vi "MultiChannelFeedbackCooling_aod_feedback(Host).vi"(5 "RIO Device":T2="RIO0") -> ()   [LabVIEW 2014]
doc: "This VI will will initialize the FPGA VI and then continually read and convert single point values from 4 channels of an analog input module."
uses:
  <vilib>/userdefined/High Color/nirio_resource_hc.ctl
  <vilib>/rvi/Analysis/host/Butterworth/config/Butterworth Filter Order.ctl
  <vilib>/rvi/Analysis/host/Butterworth/config/Butterworth Filter Type.ctl
  <vilib>/FPGAPlugInAG/PXI-7854R/niLvFpga_Open_PXI-7854R.vi
  <vilib>/FPGAPlugInAG/PXI-7854R/niLvFpga_Run_PXI-7854R.vi
  <vilib>/Utility/error.llb/Error Cluster From Error Code.vi
  <vilib>/rvi/errors/niLvFpgaAdjustHostInterfaceError.vi
  <vilib>/rvi/Analysis/host/Butterworth/config/BwScaledCoefficients.vi
  <vilib>/FPGAPlugInAG/PXI-7854R/niLvFpga_Close_PXI-7854R.vi
  <vilib>/rvi/interface/nirviOpenFPGA/nirviOpenFPGA.xnode
  FPGA Bitfiles/MultiChannelFeed_FPGATarget_MultiChannelfFee_xkdZYBc6TtU.lvbitx
  <vilib>/rvi/interface/nirviMethod/nirviMethod.xnode
  <vilib>/rvi/interface/nirviReadWriteControl/nirviReadWriteControl.xnode
  <vilib>/rvi/Analysis/host/Butterworth/XNode/ButterworthCoefficients.xnode
  <vilib>/rvi/interface/nirviCloseFPGA/nirviCloseFPGA.xnode
  <vilib>/rvi/Analysis/host/Public/NI_FpgaMspHost.lvlib
  NiFpgaLv.dll
panel:
  in  "bits per pi 2":i16=100
  in  "Reset Counter":bool
  in  "counter offset":u32
  in  "c3_delay_mult":i16=-1
  in  "c3_mult":i16=1
  in  "c2_delay_mult":i16=-1
  in  "c2_mult":i16=-1
  in  "c1_delay_mult":i16=1
  in  "c1_mult":i16=-1
  in  "c0_delay_mult":i16=1
  in  "c0_mult":i16=1
  in  "pg_img":fxp<+/-,24,12>
  in  "dg_img":fxp<+/-,24,12>
  in  "ig_img":fxp<+/-,24,6>
  in  "setpt_img":i16=3000
  in  "Upper lim_img":fxp<+/-,16,16>=1000.0
  in  "Lower lim_img":fxp<+/-,16,16>=-1000.0
  in  "output offset_img":i16
  out "Phi_filt h/lpf":dbl(graph)=-1.7364501953125
  in  "phase_hpf":dbl=2.0
  in  "Use phase hpf?":bool=TRUE
  in  "phase offset":i16
  in  "phase discont_neg":fxp<+/-,24,12>=-1.0
  in  "phase discont_pos":fxp<+/-,24,12>=1.0
  in  "Use phase lpf?":bool
  in  "phase_lpf":dbl=10000.0
  in  "Host Update Rate (msec)":dbl=1.0 format="%#_13g"
  in  "ADC Loop Timer (usec)":u32=5
  out "Phi":dbl(graph)=-0.99530029296875
  in  "Reset Phi":bool
  out "Phi Full":dbl(graph)=8.9061279296875
  in  "Bits Per Pi":i16=2000
  in  "change pars 3":bool
  in  "Mixing Level":i16=32767
  in  "Save gain setting?":bool
  in  "Step Y Gain?":bool
  in  "Enum 2":enum16{"Increase Y Gain", "Decrease Y Gain"}(ring)=enum."Decrease Y Gain"
  in  "Step X Gain?":bool
  in  "Enum":enum16{"Increase X Gain", "Decrease X Gain"}(ring)=enum."Decrease X Gain"
  in  "Ygain":T1(ring)=enum."20"
  in  "Xgain":T1(ring)=enum."20"
  in  "Change Post-Mixing Gain?":bool
  in  "Ref AOM Lvl":i16=-32768
  in  "Piezo Z":i16=-32768
  in  "power setpt":i16=7000
  in  "Upper lim pow":fxp<+/-,16,16>=10000.0
  in  "Lower lim pow":fxp<+/-,16,16>=-10000.0
  in  "hp freq pow":dbl=5000.0
  in  "lp freq pow":dbl=5000.0
  in  "Use_PID2_power":bool
  in  "hp freq 1":dbl=2200.0
  in  "hp freq 0":dbl=2200.0
  in  "lp freq 0":dbl=2200.0
  in  "DC offset 0":i16
  in  "Lower lim 0":fxp<+/-,16,16>=-1000.0
  in  "Upper lim 0":fxp<+/-,16,16>=1000.0
  in  "Dg 0":fxp<+/-,24,12>=-0.10009765625
  in  "Bead setpt 0":i16
  in  "change pars":bool
  in  "hp freq 2":dbl=1100.0
  in  "lp freq 1":dbl=2200.0
  in  "lp freq 2":dbl=1100.0
  in  "ramp power":bool
  in  "End value power":i16=1600
  in  "Step power":i16=5
  in  "Delay Time (s) power":dbl=0.01 caption="Delay Time (s)"
  in  "?":u16(ring)=2 items=["Both", "AOD", "Bead"]
  in  "?":u16(ring)=2 items=["Both", "AOD", "Bead"]
  in  "?":u16(ring) items=["Both", "AOD", "Bead"]
  in  "?":u16(ring)=2 items=["Both", "AOD", "Bead"]
  in  "?":u16(ring)=1 items=["Both", "AOD", "Bead"]
  in  "?":u16(ring)=2 items=["Both", "AOD", "Bead"]
  in  "Pg d2":fxp<+/-,24,12>=-6.0
  in  "Ig d2":fxp<+/-,24,6>=-0.7999992370605469
  in  "Dg d2":fxp<+/-,24,12>
  in  "Ig 2":fxp<+/-,24,6>
  in  "DC offset 2":i16=-16750
  in  "Lower lim 2":fxp<+/-,16,16>=-2000.0
  in  "Upper lim 2":fxp<+/-,16,16>=2000.0
  in  "Dg 2":fxp<+/-,24,12>=-1.0
  in  "Pg 2":fxp<+/-,24,12>=-0.10009765625
  in  "Bead setpt 2":i16=-2800
  in  "change pars 2":bool
  in  "change pars 1":bool
  in  "DC offset 1":i16
  in  "Lower lim 1":fxp<+/-,16,16>=-1000.0
  in  "Upper lim 1":fxp<+/-,16,16>=1000.0
  in  "Dg 1":fxp<+/-,24,12>=-0.10009765625
  in  "Bead setpt 1":i16
  out "Tot feedback + DC, Ch2":i16(graph)=-16644
  out "Individual feedback, Ch2":cluster{"fb_0":i16, "fb_d0":i16}(graph)={"fb_0"=108, "fb_d0"=108}
  out "AI2":cluster{"AI2":i16, "AI5":i16}(graph)={"AI2"=-3445, "AI5"=-3445}
  out "Tot feedback + DC, Ch1":i16(graph)=14
  out "Individual feedback, Ch1":cluster{"fb_0":i16, "fb_d0":i16}(graph)={"fb_0"=14, "fb_d0"=14}
  out "AI1":cluster{"AI1":i16, "AI4":i16}(graph)={"AI1"=1858, "AI4"=1858}
  out "Tot feedback + DC, Ch0":i16(graph)=17
  out "Individual feedback, Ch0":cluster{"fb_0":i16, "fb_d0":i16}(graph)={"fb_0"=17, "fb_d0"=17}
  out "AI0":cluster{"AI0":i16, "AI3":i16}(graph)={"AI0"=12513, "AI3"=12513}
  in  "stop":bool
  # "FPGA feedback GUI"
  # "PID controls, X (ch 0):"
  # "Gain Control"
  # "Pre-Mixing Gain"
  # "Ref Mixing Level"
  # "PID controls, Y (ch 1):"
  # "Bead feedback:"
  # "Post-Mixing Gain"
  # "Backscatter Interferometer Settings"
  # "Phase wrapping"
  # "Bead feedback:"
  # "PID controls, Z (ch 2):"
  # "Bead feedback:"
  # "AOD feeback:"
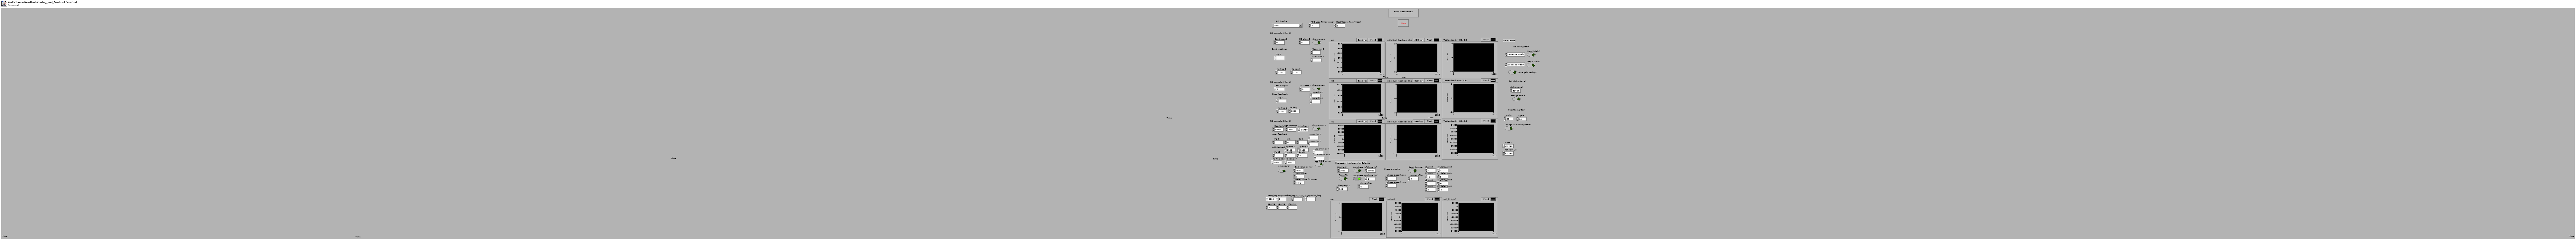
[diagram p1: front panel]
types:
  T1 = enum16{"1", "2", "4", "8", "10", "20", "40", "80", "100", "200", "400", "800"}
  T2 = typedef "nirio_resource_hc.ctl" = tag
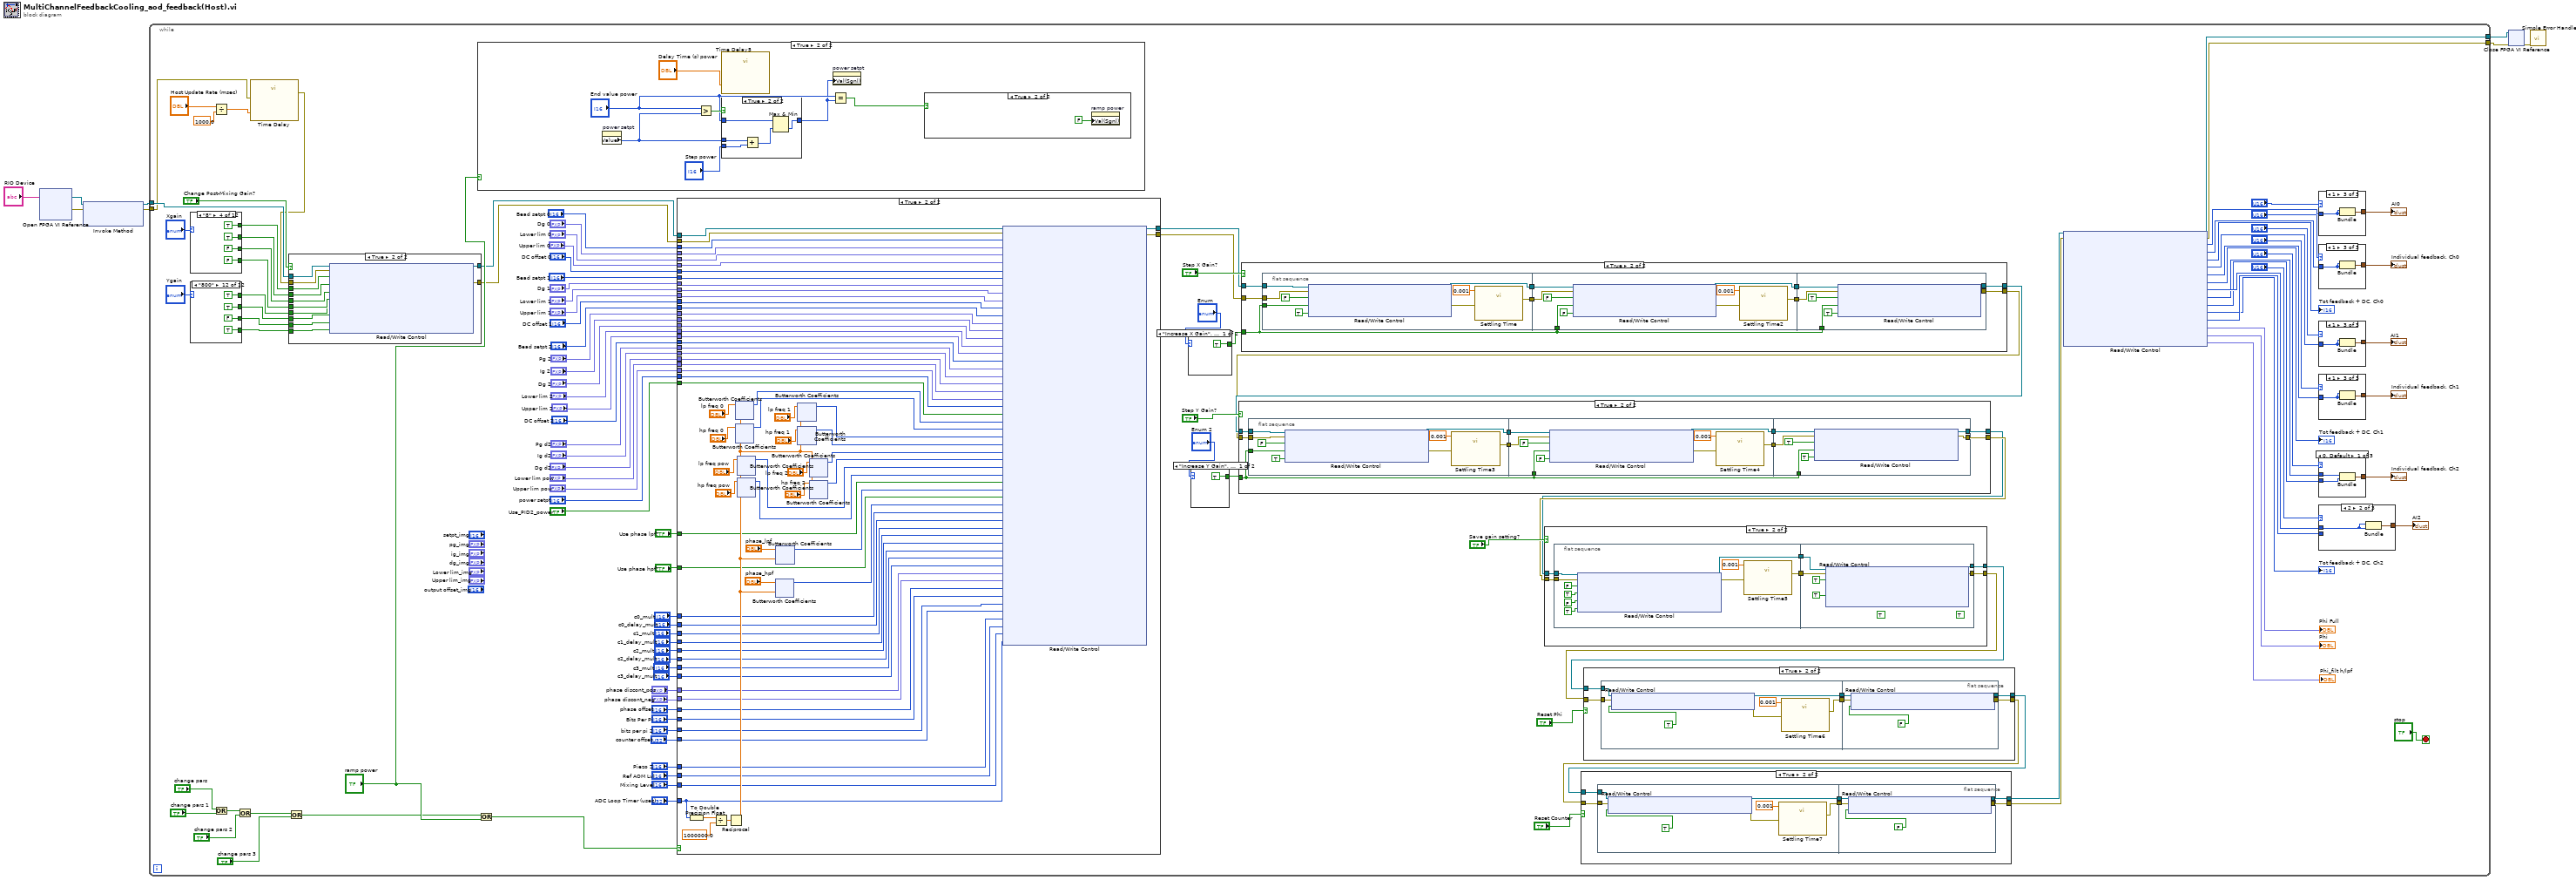
[diagram p0: block diagram]
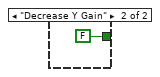
[diagram p6: hidden frame]
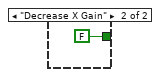
[diagram p8: hidden frame]
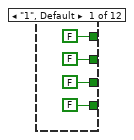
[diagram p9: hidden frame]
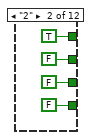
[diagram p10: hidden frame]
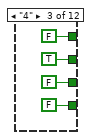
[diagram p11: hidden frame]
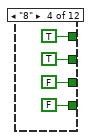
[diagram p12: hidden frame]
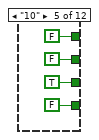
[diagram p13: hidden frame]
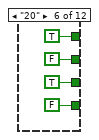
[diagram p14: hidden frame]
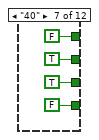
[diagram p15: hidden frame]
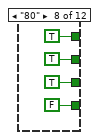
[diagram p16: hidden frame]
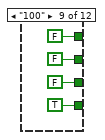
[diagram p17: hidden frame]
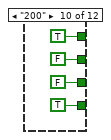
[diagram p18: hidden frame]
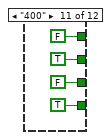
[diagram p19: hidden frame]
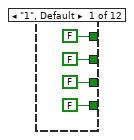
[diagram p20: hidden frame]
diagram:
  n1 = xnode "Open FPGA VI Reference"("resource name"="RIO Device") -> ("FPGA VI Reference Out"=w3:refnum<k20>, "error out"=w2:errorcluster)  [unwired: 1 in]
  n2 = xnode "Invoke Method"("FPGA VI Reference In"=w3, "error in"=w2) -> ("FPGA VI Reference Out"=w5:refnum<k20>, "error out"=w4:errorcluster)  [unwired: 1 in]
  n3 = while {
    tunnel: [w130] -> w8
    tunnel: w5 -> [w61]
    tunnel: w4 -> [w32]
    tunnel: [w129] -> w1
    stop <- "stop" stop-if-true
    n4 = case shown="\"8\"" "Xgain" {
      tunnel: [FALSE TRUE FALSE TRUE FALSE TRUE FALSE TRUE FALSE TRUE FALSE TRUE] -> w71
      tunnel: [FALSE FALSE TRUE TRUE FALSE FALSE TRUE TRUE FALSE FALSE TRUE TRUE] -> w70
      tunnel: [FALSE FALSE FALSE FALSE TRUE TRUE TRUE TRUE FALSE FALSE FALSE FALSE] -> w69
      tunnel: [FALSE FALSE FALSE FALSE FALSE FALSE FALSE FALSE TRUE TRUE TRUE TRUE] -> w68
      frame "1", Default {
      }
      frame "2" {
      }
      frame "4" {
      }
      frame "8" {
      }
      frame "10" {
      }
      frame "20" {
      }
      frame "40" {
      }
      frame "80" {
      }
      frame "100" {
      }
      frame "200" {
      }
      frame "400" {
      }
      frame "800" {
      }
    }
    n5 = case shown="\"800\"" "Ygain" {
      tunnel: [FALSE TRUE FALSE TRUE FALSE TRUE FALSE TRUE FALSE TRUE FALSE TRUE] -> w63
      tunnel: [FALSE FALSE TRUE TRUE FALSE FALSE TRUE TRUE FALSE FALSE TRUE TRUE] -> w64
      tunnel: [FALSE FALSE FALSE FALSE TRUE TRUE TRUE TRUE FALSE FALSE FALSE FALSE] -> w65
      tunnel: [FALSE FALSE FALSE FALSE FALSE FALSE FALSE FALSE TRUE TRUE TRUE TRUE] -> w66
      frame "1", Default {
      }
      frame "2" {
      }
      frame "4" {
      }
      frame "8" {
      }
      frame "10" {
      }
      frame "20" {
      }
      frame "40" {
      }
      frame "80" {
      }
      frame "100" {
      }
      frame "200" {
      }
      frame "400" {
      }
      frame "800" {
      }
    }
    n6 = Divide(x="Host Update Rate (msec)", y=1000.0) -> (x/y=w34:dbl)
    n7 = Or(x="change pars", y="change pars 1") -> (x .or. y?=w104:bool)
    n8 = Or(x=w104, y="change pars 2") -> (x .or. y?=w43:bool)
    n9 = call "Time Delay"("error in (no error)"=w32, "Delay Time (s)"=w34) -> ("error out"=w31:errorcluster)  [unwired: 9 in]
    n10 = case shown="True" "Change Post-Mixing Gain?" {
      tunnel: w71 -> [_ w380]
      tunnel: w70 -> [_ w379]
      tunnel: w69 -> [_ w378]
      tunnel: w68 -> [_ w377]
      tunnel: w66 -> [_ w376]
      tunnel: w65 -> [_ w375]
      tunnel: w64 -> [_ w374]
      tunnel: w63 -> [_ w373]
      tunnel: w31 -> [w367 w372]
      tunnel: [w367 w371] -> w62
      tunnel: w61 -> [w368 w370]
      tunnel: [w368 w369] -> w60
      frame False {
      }
      frame True {
        n11 = xnode "Read/Write Control"("FPGA VI Reference In"=w370, "error in"=w372, "XD0"=w380, "XD1"=w379, "XD2"=w378, "XD3"=w377, "YD0"=w373, "YD1"=w374, "YD2"=w375, "YD3"=w376) -> ("FPGA VI Reference Out"=w369:refnum<k20>, "error out"=w371:errorcluster)
      }
    }
    n12 = Or(x=w43, y="change pars 3") -> (x .or. y?=w30:bool)
    n13 = case shown="True" "ramp power" {
      frame False {
      }
      frame True {
        n14 = property on="power setpt" class="DigNum (strict)"() -> ("Value"=w382:i16)  [unwired: 2 in, 2 out]
        n15 = Greater?(x="End value power", y=w382) -> (0:w387:bool)
        n16 = call "Time Delay5"("Delay Time (s)"="Delay Time (s) power") -> ()  [unwired: 10 in, 1 out]
        n17 = case shown="True" w387 {
          tunnel: "End value power" -> [w390 w395]
          tunnel: w382 -> [w393 w398]
          tunnel: "Step power" -> [w392 w397]
          tunnel: [w389 w394] -> w381
          frame False {
            n18 = Subtract(x=w393, y=w392) -> (x-y=w391:i16)
            n19 = Max & Min(x=w390, y=w391) -> (max(x,y)=w389:i16)  [unwired: 1 out]
          }
          frame True {
            n20 = Add(x=w398, y=w397) -> (x+y=w396:i16)
            n21 = Max & Min(x=w395, y=w396) -> (min(x,y)=w394:i16)  [unwired: 1 out]
          }
        }
        n22 = property on="power setpt" class="DigNum (strict)"("Val(Sgnl)"=w381) -> ()  [unwired: 2 in, 2 out]
        n23 = Equal?(x="End value power", y=w381) -> (x = y?=w386:bool)
        n24 = case shown="True" w386 {
          frame False {
          }
          frame True {
            n25 = property on="ramp power" class="Bool (strict)"("Val(Sgnl)"=FALSE) -> ()  [unwired: 2 in, 2 out]
          }
        }
      }
    }
    n26 = Or(x=w30, y="ramp power") -> (x .or. y?=w80:bool)
    n27 = case shown="True" w80 {
      tunnel: w62 -> [w438 w502]
      tunnel: [w438 w510] -> w49
      tunnel: [w437 w509] -> w50
      tunnel: "Bead setpt 0" -> [_ w508]
      tunnel: "Dg 0" -> [_ w507]
      tunnel: "Upper lim 0" -> [_ w505]
      tunnel: "Lower lim 0" -> [_ w506]
      tunnel: "DC offset 0" -> [_ w504]
      tunnel: w60 -> [w437 w503]
      tunnel: "Bead setpt 1" -> [_ w501]
      tunnel: "Dg 1" -> [_ w500]
      tunnel: "Lower lim 1" -> [_ w499]
      tunnel: "Upper lim 1" -> [_ w498]
      tunnel: "DC offset 1" -> [_ w475]
      tunnel: "Bead setpt 2" -> [_ w497]
      tunnel: "Pg 2" -> [_ w496]
      tunnel: "Ig 2" -> [_ w477]
      tunnel: "Dg 2" -> [_ w495]
      tunnel: "Lower lim 2" -> [_ w494]
      tunnel: "Upper lim 2" -> [_ w493]
      tunnel: "DC offset 2" -> [_ w492]
      tunnel: "Pg d2" -> [_ w476]
      tunnel: "Ig d2" -> [_ w482]
      tunnel: "Dg d2" -> [_ w481]
      tunnel: "Use_PID2_power" -> [_ w485]
      tunnel: "Lower lim pow" -> [_ w478]
      tunnel: "Upper lim pow" -> [_ w479]
      tunnel: "power setpt" -> [_ w480]
      tunnel: "Piezo Z" -> [_ w453]
      tunnel: "Ref AOM Lvl" -> [_ w454]
      tunnel: "Mixing Level" -> [_ w455]
      tunnel: "Bits Per Pi" -> [_ w441]
      tunnel: "ADC Loop Timer (usec)" -> [_ w456]
      tunnel: "Use phase lpf?" -> [_ w460]
      tunnel: "phase discont_pos" -> [_ w444]
      tunnel: "phase discont_neg" -> [_ w443]
      tunnel: "phase offset" -> [_ w442]
      tunnel: "Use phase hpf?" -> [_ w458]
      tunnel: "c0_mult" -> [_ w452]
      tunnel: "c0_delay_mult" -> [_ w451]
      tunnel: "c1_mult" -> [_ w450]
      tunnel: "c1_delay_mult" -> [_ w449]
      tunnel: "c2_mult" -> [_ w448]
      tunnel: "c2_delay_mult" -> [_ w447]
      tunnel: "c3_mult" -> [_ w446]
      tunnel: "c3_delay_mult" -> [_ w445]
      tunnel: "counter offset" -> [_ w440]
      tunnel: "bits per pi 2" -> [_ w439]
      frame False {
      }
      frame True {
        n28 = To Double Precision Float(number=w456) -> (double precision float=w466:dbl)
        n29 = Divide(x=w466, y=1000000.0) -> (x/y=w464:dbl)
        n30 = Reciprocal(x=w464) -> (1/x=w463:dbl)
        n31 = xnode "Butterworth Coefficients"("cutoff frequency (Hz)"="lp freq 0", "sample rate (S/s)"=w463) -> ("scaled coefficients"=w474:i32[])  [unwired: 1 in, 1 out]
        n32 = xnode "Butterworth Coefficients"("cutoff frequency (Hz)"="hp freq 0", "sample rate (S/s)"=w463) -> ("scaled coefficients"=w473:i32[])  [unwired: 1 in, 1 out]
        n33 = xnode "Butterworth Coefficients"("cutoff frequency (Hz)"="lp freq pow", "sample rate (S/s)"=w463) -> ("scaled coefficients"=w467:i32[])  [unwired: 1 in, 1 out]
        n34 = xnode "Butterworth Coefficients"("cutoff frequency (Hz)"="hp freq pow", "sample rate (S/s)"=w463) -> ("scaled coefficients"=w468:i32[])  [unwired: 1 in, 1 out]
        n35 = xnode "Butterworth Coefficients"("cutoff frequency (Hz)"="phase_hpf", "sample rate (S/s)"=w463) -> ("scaled coefficients"=w457:i32[])  [unwired: 1 in, 1 out]
        n36 = xnode "Butterworth Coefficients"("cutoff frequency (Hz)"="phase_lpf", "sample rate (S/s)"=w463) -> ("scaled coefficients"=w459:i32[])  [unwired: 1 in, 1 out]
        n37 = xnode "Butterworth Coefficients"("cutoff frequency (Hz)"="lp freq 1", "sample rate (S/s)"=w463) -> ("scaled coefficients"=w472:i32[])  [unwired: 1 in, 1 out]
        n38 = xnode "Butterworth Coefficients"("cutoff frequency (Hz)"="hp freq 1", "sample rate (S/s)"=w463) -> ("scaled coefficients"=w471:i32[])  [unwired: 1 in, 1 out]
        n39 = xnode "Butterworth Coefficients"("cutoff frequency (Hz)"="lp freq 2", "sample rate (S/s)"=w463) -> ("scaled coefficients"=w470:i32[])  [unwired: 1 in, 1 out]
        n40 = xnode "Butterworth Coefficients"("cutoff frequency (Hz)"="hp freq 2", "sample rate (S/s)"=w463) -> ("scaled coefficients"=w469:i32[])  [unwired: 1 in, 1 out]
        n41 = xnode "Read/Write Control"("FPGA VI Reference In"=w503, "error in"=w502, "Dc Pos 0"=w508, "dg 0"=w507, "Lower lim 0"=w506, "Upper lim 0"=w505, "output offset 0"=w504, "Dc Pos 1"=w501, "dg 1"=w500, "Lower lim 1"=w499, "Upper lim 1"=w498, "output offset 1"=w475, "Dc Pos 2"=w497, "pg 2"=w496, "ig 3"=w477, "dg 2"=w495, "Lower lim 2"=w494, "Upper lim 2"=w493, "output offset 2"=w492, "pg pow"=w476, "ig pow"=w482, "dg pow"=w481, "Lower lim pow"=w478, "Upper lim pow"=w479, "Dc Pos pow"=w480, "Use_PID2_X 2"=w485, "lp coeff 0"=w474, "hp coeff 0"=w473, "lp coeff 1"=w472, "hp coeff 1"=w471, "lp coeff 2"=w470, "hp coeff 2"=w469, "lp coeff pow"=w467, "hp coeff pow"=w468, "use lpf?"=w460, "phase_lpf coeff"=w459, "use hpf?"=w458, "phase_hpf coeff"=w457, "c0_mult"=w452, "c0_delay_mult"=w451, "c1_mult"=w450, "c1_delay_mult"=w449, "c2_mult"=w448, "c2_delay_mult"=w447, "c3_mult"=w446, "c3_delay_mult"=w445, "discont_pos"=w444, "discont_neg"=w443, "phase offset"=w442, "bits per pi"=w441, "bits per pi 2"=w439, "Counter Offset"=w440, "Piezo Z"=w453, "Ref AOM Lvl"=w454, "Mixing Level"=w455, "loop timer (usec)"=w456) -> ("FPGA VI Reference Out"=w509:refnum<k20>, "error out"=w510:errorcluster)
      }
    }
    n42 = case shown="\"Increase X Gain\", Default" "Enum" {
      tunnel: [TRUE FALSE] -> w56
      frame "Increase X Gain", Default {
      }
      frame "Decrease X Gain" {
      }
    }
    n43 = case shown="\"Increase Y Gain\", Default" "Enum 2" {
      tunnel: [TRUE FALSE] -> w53
      frame "Increase Y Gain", Default {
      }
      frame "Decrease Y Gain" {
      }
    }
    n44 = case shown="True" "Step X Gain?" {
      tunnel: w56 -> [_ w243]
      tunnel: [w234 w238] -> w52
      tunnel: [w233 w237] -> w51
      tunnel: w50 -> [w234 w236]
      tunnel: w49 -> [w233 w235]
      frame False {
      }
      frame True {
        n45 = flat-sequence {
          tunnel: w243 -> [w252]
          tunnel: [w247] -> w242
          tunnel: [w246] -> w240
          tunnel: w236 -> [w245]
          tunnel: w235 -> [w244]
          tunnel: w243 -> [w261]
          tunnel: w242 -> [w257]
          tunnel: [w255] -> w241
          tunnel: w240 -> [w254]
          tunnel: [w253] -> w239
          tunnel: w243 -> [w268]
          tunnel: w241 -> [w265]
          tunnel: w239 -> [w264]
          tunnel: [w263] -> w238
          tunnel: [w262] -> w237
          frame #0 {
            n46 = xnode "Read/Write Control"("FPGA VI Reference In"=w245, "error in"=w244, "Xen"=FALSE, "Xud"=w252, "Xinc"=TRUE) -> ("FPGA VI Reference Out"=w246:refnum<k20>, "error out"=w248:errorcluster)
            n47 = call "Settling Time"("error in (no error)"=w248, "Delay Time (s)"=0.001) -> ("error out"=w247:errorcluster)  [unwired: 9 in]
          }
          frame #1 {
            n48 = xnode "Read/Write Control"("FPGA VI Reference In"=w254, "error in"=w257, "Xen"=FALSE, "Xud"=w261, "Xinc"=FALSE) -> ("FPGA VI Reference Out"=w253:refnum<k20>, "error out"=w256:errorcluster)
            n49 = call "Settling Time2"("error in (no error)"=w256, "Delay Time (s)"=0.001) -> ("error out"=w255:errorcluster)  [unwired: 9 in]
          }
          frame #2 {
            n50 = xnode "Read/Write Control"("FPGA VI Reference In"=w264, "error in"=w265, "Xen"=TRUE, "Xud"=w268, "Xinc"=TRUE) -> ("FPGA VI Reference Out"=w263:refnum<k20>, "error out"=w262:errorcluster)
          }
        }
      }
    }
    n51 = case shown="True" "Step Y Gain?" {
      tunnel: w53 -> [_ w205]
      tunnel: w52 -> [w196 w200]
      tunnel: w51 -> [w195 w199]
      tunnel: [w196 w198] -> w46
      tunnel: [w195 w197] -> w47
      frame False {
      }
      frame True {
        n52 = flat-sequence {
          tunnel: w205 -> [w214]
          tunnel: [w209] -> w204
          tunnel: [w208] -> w202
          tunnel: w200 -> [w207]
          tunnel: w199 -> [w206]
          tunnel: w205 -> [w223]
          tunnel: w204 -> [w219]
          tunnel: [w217] -> w203
          tunnel: w202 -> [w216]
          tunnel: [w215] -> w201
          tunnel: w205 -> [w230]
          tunnel: w203 -> [w227]
          tunnel: w201 -> [w226]
          tunnel: [w225] -> w198
          tunnel: [w224] -> w197
          frame #0 {
            n53 = xnode "Read/Write Control"("FPGA VI Reference In"=w207, "error in"=w206, "Yen"=FALSE, "Yud"=w214, "Yinc"=TRUE) -> ("FPGA VI Reference Out"=w208:refnum<k20>, "error out"=w210:errorcluster)
            n54 = call "Settling Time3"("error in (no error)"=w210, "Delay Time (s)"=0.001) -> ("error out"=w209:errorcluster)  [unwired: 9 in]
          }
          frame #1 {
            n55 = xnode "Read/Write Control"("FPGA VI Reference In"=w216, "error in"=w219, "Yen"=FALSE, "Yud"=w223, "Yinc"=FALSE) -> ("FPGA VI Reference Out"=w215:refnum<k20>, "error out"=w218:errorcluster)
            n56 = call "Settling Time4"("error in (no error)"=w218, "Delay Time (s)"=0.001) -> ("error out"=w217:errorcluster)  [unwired: 9 in]
          }
          frame #2 {
            n57 = xnode "Read/Write Control"("FPGA VI Reference In"=w226, "error in"=w227, "Yen"=TRUE, "Yud"=w230, "Yinc"=TRUE) -> ("FPGA VI Reference Out"=w225:refnum<k20>, "error out"=w224:errorcluster)
          }
        }
      }
    }
    n58 = case shown="True" "Save gain setting?" {
      tunnel: w46 -> [w172 w173]
      tunnel: w47 -> [w171 w176]
      tunnel: [w172 w175] -> w40
      tunnel: [w171 w174] -> w38
      frame False {
      }
      frame True {
        n59 = flat-sequence {
          tunnel: [w184] -> w178
          tunnel: [w183] -> w177
          tunnel: w176 -> [w182]
          tunnel: w173 -> [w179]
          tunnel: w178 -> [w192]
          tunnel: w177 -> [w191]
          tunnel: [w190] -> w175
          tunnel: [w189] -> w174
          frame #0 {
            n60 = xnode "Read/Write Control"("FPGA VI Reference In"=w179, "error in"=w182, "Yen"=FALSE, "Yinc"=TRUE, "Xen"=FALSE, "Xinc"=TRUE) -> ("FPGA VI Reference Out"=w183:refnum<k20>, "error out"=w185:errorcluster)
            n61 = call "Settling Time5"("error in (no error)"=w185, "Delay Time (s)"=0.001) -> ("error out"=w184:errorcluster)  [unwired: 9 in]
          }
          frame #1 {
            (unwired) TRUE
            (unwired) TRUE
            n62 = xnode "Read/Write Control"("FPGA VI Reference In"=w191, "error in"=w192, "Yen"=TRUE, "Xen"=TRUE) -> ("FPGA VI Reference Out"=w190:refnum<k20>, "error out"=w189:errorcluster)  [unwired: 2 in]
          }
        }
      }
    }
    n63 = case shown="True" "Reset Phi" {
      tunnel: w40 -> [w152 w158]
      tunnel: w38 -> [w151 w157]
      tunnel: [w152 w153] -> w12
      tunnel: [w151 w154] -> w13
      frame False {
      }
      frame True {
        n64 = flat-sequence {
          tunnel: w158 -> [w165]
          tunnel: w157 -> [w164]
          tunnel: [w163] -> w156
          tunnel: [w159] -> w155
          tunnel: w156 -> [w170]
          tunnel: w155 -> [w169]
          tunnel: [w167] -> w153
          tunnel: [w166] -> w154
          frame #0 {
            n65 = xnode "Read/Write Control"("FPGA VI Reference In"=w165, "error in"=w164, "Reset Phi"=TRUE) -> ("FPGA VI Reference Out"=w163:refnum<k20>, "error out"=w160:errorcluster)
            n66 = call "Settling Time6"("error in (no error)"=w160, "Delay Time (s)"=0.001) -> ("error out"=w159:errorcluster)  [unwired: 9 in]
          }
          frame #1 {
            n67 = xnode "Read/Write Control"("FPGA VI Reference In"=w170, "error in"=w169, "Reset Phi"=FALSE) -> ("FPGA VI Reference Out"=w167:refnum<k20>, "error out"=w166:errorcluster)
          }
        }
      }
    }
    n68 = case shown="True" "Reset Counter" {
      tunnel: w12 -> [w132 w138]
      tunnel: w13 -> [w131 w137]
      tunnel: [w132 w134] -> w11
      tunnel: [w131 w133] -> w10
      frame False {
      }
      frame True {
        n69 = flat-sequence {
          tunnel: w138 -> [w145]
          tunnel: w137 -> [w144]
          tunnel: [w143] -> w136
          tunnel: [w139] -> w135
          tunnel: w136 -> [w150]
          tunnel: w135 -> [w149]
          tunnel: [w147] -> w134
          tunnel: [w146] -> w133
          frame #0 {
            n70 = xnode "Read/Write Control"("FPGA VI Reference In"=w145, "error in"=w144, "Reset Counter"=TRUE) -> ("FPGA VI Reference Out"=w143:refnum<k20>, "error out"=w140:errorcluster)
            n71 = call "Settling Time7"("error in (no error)"=w140, "Delay Time (s)"=0.001) -> ("error out"=w139:errorcluster)  [unwired: 9 in]
          }
          frame #1 {
            n72 = xnode "Read/Write Control"("FPGA VI Reference In"=w150, "error in"=w149, "Reset Counter"=FALSE) -> ("FPGA VI Reference Out"=w147:refnum<k20>, "error out"=w146:errorcluster)
          }
        }
      }
    }
    n73 = xnode "Read/Write Control"("FPGA VI Reference In"=w11, "error in"=w10) -> ("FPGA VI Reference Out"=w130:refnum<k20>, "error out"=w129:errorcluster, "AI0"=w103:i16, "fb_0"=w98:i16, "tot_fb_0"=→"Tot feedback + DC, Ch0":i16, "AI1"=w95:i16, "fb_1"=w93:i16, "tot_fb_1"=→"Tot feedback + DC, Ch1":i16, "AI2"=w90:i16, "fb_2"=w86:i16, "fb_d2"=w85:i16, "tot_fb_2"=→"Tot feedback + DC, Ch2":i16, "AI5"=w87:i16, "Phi Full"=→"Phi Full":fxp<+/-,32,18>, "Phi"=→"Phi":fxp<+/-,16,2>, "Phi Full h/lpf"=→"Phi_filt h/lpf":fxp<+/-,36,22>)
    n74 = case shown="1" "?" {
      tunnel: w103 -> [w432 w433 w436]
      tunnel: [w431 w434 w435] -> w102
      frame 0, Default {
        n75 = Bundle("AI0"=w432, "AI0"=w432) -> (w431:cluster{"AI0":i16, "AI0":i16})  [unwired: 1 in]
      }
      frame 2 {
        n76 = Bundle("AI0"=w433, "AI0"=w433) -> (w434:cluster{"AI0":i16, "AI0":i16})  [unwired: 1 in]
      }
      frame 1 {
        n77 = Bundle("AI0"=w436, "AI0"=w436) -> (w435:cluster{"AI0":i16, "AI0":i16})  [unwired: 1 in]
      }
    }
    "AI0" <- w102
    n78 = case shown="1" "?" {
      tunnel: w98 -> [w426 w427 w430]
      tunnel: [w425 w428 w429] -> w100
      frame 0, Default {
        n79 = Bundle("fb_0"=w426, "fb_0"=w426) -> (w425:cluster{"fb_0":i16, "fb_0":i16})  [unwired: 1 in]
      }
      frame 2 {
        n80 = Bundle("fb_0"=w427, "fb_0"=w427) -> (w428:cluster{"fb_0":i16, "fb_0":i16})  [unwired: 1 in]
      }
      frame 1 {
        n81 = Bundle("fb_0"=w430, "fb_0"=w430) -> (w429:cluster{"fb_0":i16, "fb_0":i16})  [unwired: 1 in]
      }
    }
    "Individual feedback, Ch0" <- w100
    n82 = case shown="1" "?" {
      tunnel: w95 -> [w419 w421 w423]
      tunnel: [w420 w422 w424] -> w81
      frame 0, Default {
        n83 = Bundle("AI1"=w419, "AI1"=w419) -> (w420:cluster{"AI1":i16, "AI1":i16})  [unwired: 1 in]
      }
      frame 2 {
        n84 = Bundle("AI1"=w421, "AI1"=w421) -> (w422:cluster{"AI1":i16, "AI1":i16})  [unwired: 1 in]
      }
      frame 1 {
        n85 = Bundle("AI1"=w423, "AI1"=w423) -> (w424:cluster{"AI1":i16, "AI1":i16})  [unwired: 1 in]
      }
    }
    "AI1" <- w81
    n86 = case shown="1" "?" {
      tunnel: w93 -> [w413 w415 w418]
      tunnel: [w414 w416 w417] -> w92
      frame 0, Default {
        n87 = Bundle("fb_1"=w413, "fb_1"=w413) -> (w414:cluster{"fb_1":i16, "fb_1":i16})  [unwired: 1 in]
      }
      frame 2 {
        n88 = Bundle("fb_1"=w415, "fb_1"=w415) -> (w416:cluster{"fb_1":i16, "fb_1":i16})  [unwired: 1 in]
      }
      frame 1 {
        n89 = Bundle("fb_1"=w418, "fb_1"=w418) -> (w417:cluster{"fb_1":i16, "fb_1":i16})  [unwired: 1 in]
      }
    }
    "Individual feedback, Ch1" <- w92
    n90 = case shown="0, Default" "?" {
      tunnel: w86 -> [w401 w402 _]
      tunnel: w85 -> [w400 _ w405]
      tunnel: [w399 w403 w404] -> w83
      frame 0, Default {
        n91 = Bundle("fb_2"=w401, "fb_d2"=w400) -> (w399:cluster{"fb_2":i16, "fb_d2":i16})  [unwired: 1 in]
      }
      frame 2 {
        n92 = Bundle("fb_2"=w402, "fb_2"=w402) -> (w403:cluster{"fb_2":i16, "fb_2":i16})  [unwired: 1 in]
      }
      frame 1 {
        n93 = Bundle("fb_d2"=w405, "fb_d2"=w405) -> (w404:cluster{"fb_d2":i16, "fb_d2":i16})  [unwired: 1 in]
      }
    }
    "Individual feedback, Ch2" <- w83
    n94 = case shown="2" "?" {
      tunnel: w90 -> [w408 w409 _]
      tunnel: w87 -> [w407 _ w412]
      tunnel: [w406 w410 w411] -> w82
      frame 0, Default {
        n95 = Bundle("AI2"=w408, "AI5"=w407) -> (w406:cluster{"AI2":i16, "AI5":i16})  [unwired: 1 in]
      }
      frame 2 {
        n96 = Bundle("AI2"=w409, "AI2"=w409) -> (w410:cluster{"AI2":i16, "AI2":i16})  [unwired: 1 in]
      }
      frame 1 {
        n97 = Bundle("AI5"=w412, "AI5"=w412) -> (w411:cluster{"AI5":i16, "AI5":i16})  [unwired: 1 in]
      }
    }
    "AI2" <- w82
  }
  n98 = xnode "Close FPGA VI Reference"("FPGA VI Reference In"=w8, "error in"=w1) -> ("error out"=w7:errorcluster)
  n99 = call <vilib>:"Simple Error Handler.vi"("error in (no error)"=w7) -> ()  [unwired: 4 in, 5 out]
